vi "Call Function with Shared Variable.vi"(8 "error in (no error)":errorcluster, 11 "Python Driver in":refnum<class "Python Driver.lvclass">) -> (0 "error out":errorcluster, 3 "Python Driver out":refnum<class "Python Driver.lvclass">)   [LabVIEW 2022 SP3, in "Python Driver.lvclass"]
uses:
  Python Driver.lvclass
  Python Driver.lvclass/Python Driver.ctl
panel:
  out "standard error":string
  out "standard output":string
  in  "Fetch":bool
  in  "stop":bool
  out "Weather":dbl[](array[numeric])
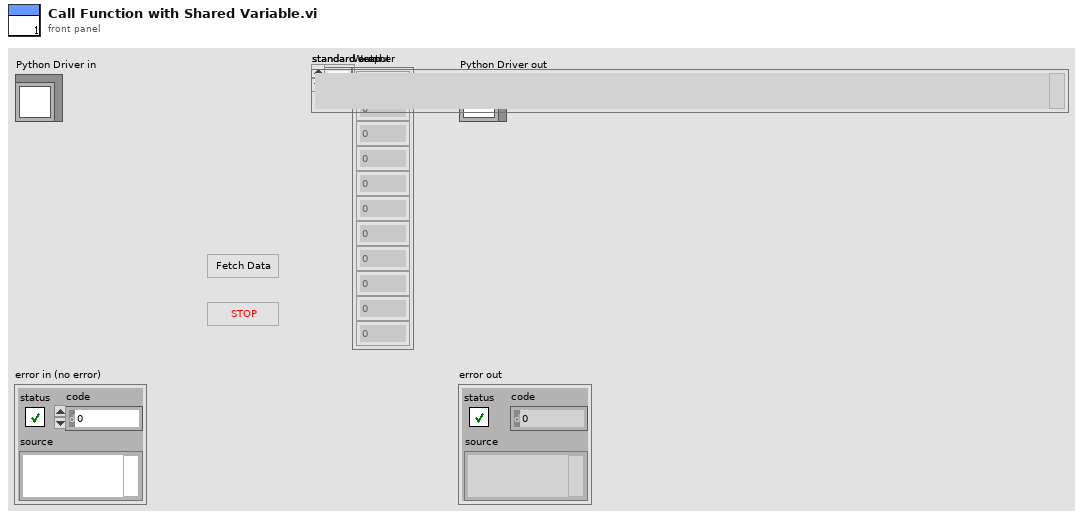
[diagram p1: front panel]
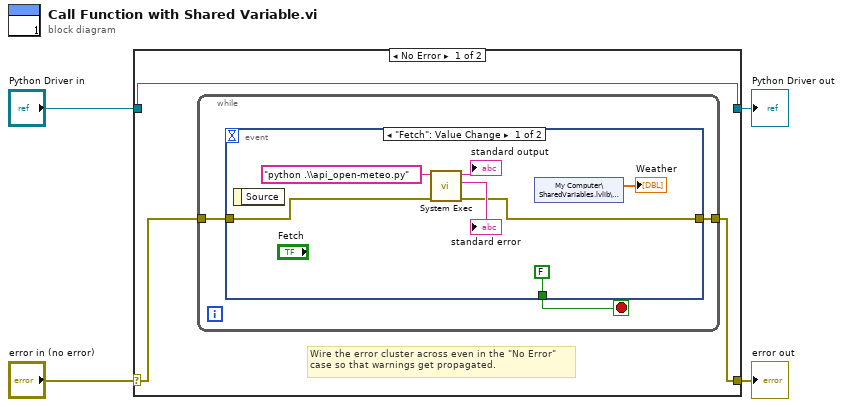
[diagram p0: block diagram]
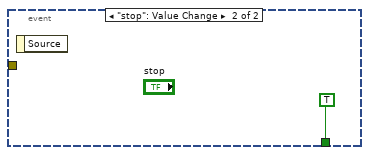
[diagram p2: hidden frame]
diagram:
  n1 = case shown="No Error" "error in (no error)" {
    selector: "error in (no error)" -> [w6 w20]
    tunnel: [w5 w20] -> w3
    tunnel: [w7 w19] -> w1
    tunnel: "Python Driver in" -> [w7 w19]
    frame No Error {
      # "Wire the error cluster across even in the \"No Error\"\ncase so that warnings get propagated."
      n2 = while {
        tunnel: w6 -> [w9]
        tunnel: [w8] -> w5
        stop <- w10 stop-if-true
        n3 = event shown="[0] \"Fetch\": Value Change" {
          selector: _ -> [_ _]
          dyn-events: _ -> [_ _]
          timeout: _ -> [_ _]
          tunnel: [FALSE ("stop") TRUE ("stop")] -> w10
          tunnel: w9 -> [w12 _]
          tunnel: [w11 _] -> w8
          event "Fetch": Value Change {
            n4 = event-data() -> ()  [unwired: 1 in, 1 out]
            n5 = call <vilib>:"System Exec.vi"("error in (no error)"=w12, "command line"="python .\\api_open-meteo.py") -> ("error out"=w11:errorcluster, "standard error"=→"standard error":string, "standard output"=→"standard output":string)  [unwired: 6 in, 1 out]
            n6 = shared-variable "My Computer\\SharedVariables.lvlib\\Weather"() -> (→"Weather":dbl[])  [unwired: 1 in, 1 out]
          }
          event "stop": Value Change {
            n7 = event-data() -> ()  [unwired: 1 in, 1 out]
          }
        }
      }
    }
    frame Error {
    }
  }
  "error out" <- w3
  "Python Driver out" <- w1
